vi "Configure Trigger (I2C - Address Or Data).vi"(0 "VISA resource name":refnum<visa-resource-name>, 1 "Trigger On (4:Address)":u16(ring)=4 items=["Address"=4, "Data"=5, "Address And Data"=6], 2 "Addressing Mode (0:7 Bit)":u16(ring) items=["7 Bit", "10 Bit"], 3 "Special Address (0:None)":u16(ring) items=["None", "Start", "General Call", "10 Bit"], 5 "Data Source":T2={"Data Source (0:Channel1)"=0, "Data Threshold (1.2V)"=1.2} {"Data Source (0:Channel1)" items=["Channel1", "Channel2", "Channel3", "Channel4"]}, 7 "Clock Source":T1={"Clock Source (1:Channel2) "=1, "Clock Threshold (1.2V)"=1.2} {"Clock Source (1:Channel2)" items=["Channel1", "Channel2", "Channel3", "Channel4"]}, 9 "Data Direction (0:Either)":u16(ring) items=["Either", "Read", "Write"], 11 "error in (no error)":errorcluster, 12 "Address Value":string, 13 "Data Start Position(0)":u16, 14 "Data Value":string) -> (4 "VISA resource name out":refnum<visa-resource-name>, 15 "error out":errorcluster)   [LabVIEW 2015, in "Tektronix 7000 Series.lvlib"]
doc: "Configures I2C trigger settings for an oscilloscope. A trigger occurs when an Inter-IC Control signal is found. This Vi is configure trigger on Address,Data, Address And Data\n\n<b>Note:</b>\nOnly DPO7000 series oscilloscopes Support this Trigger."
uses:
  <instrlib>/Tektronix 7000 Series/Tektronix 7000 Series.lvlib
panel:
  # "lsb"
  # "msb"
  # "msb"
  # "lsb"
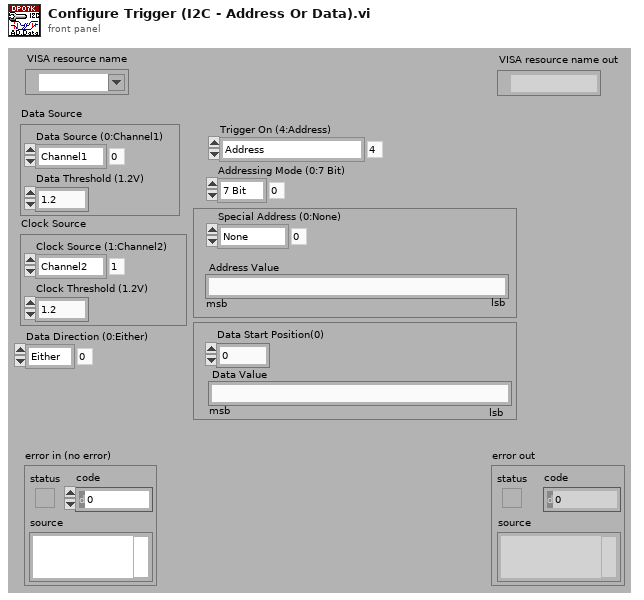
[diagram p1: front panel]
types:
  T1 = cluster{"Clock Source (1:Channel2) ":u16, "Clock Threshold (1.2V)":dbl}
  T2 = cluster{"Data Source (0:Channel1)":u16, "Data Threshold (1.2V)":dbl}
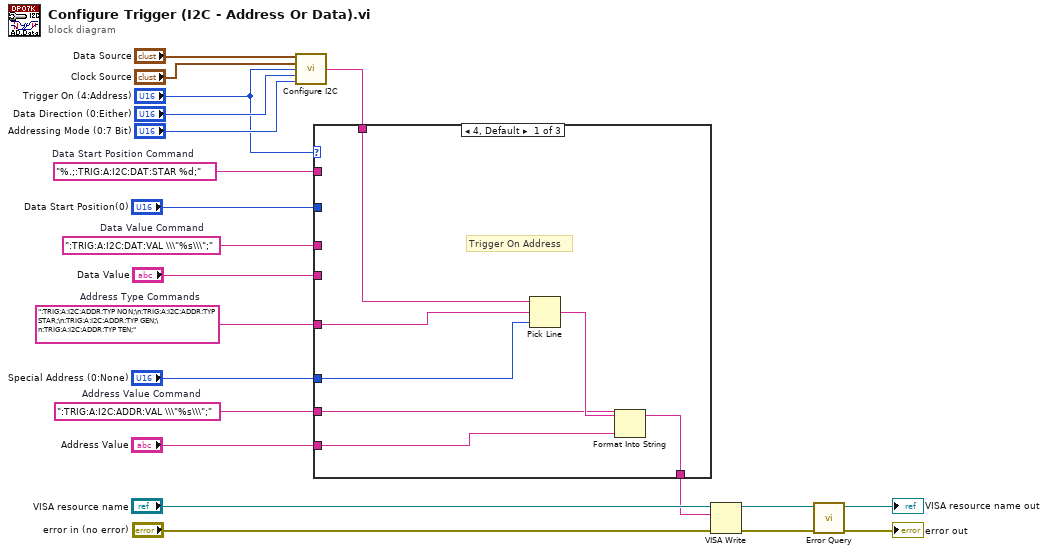
[diagram p0: block diagram]
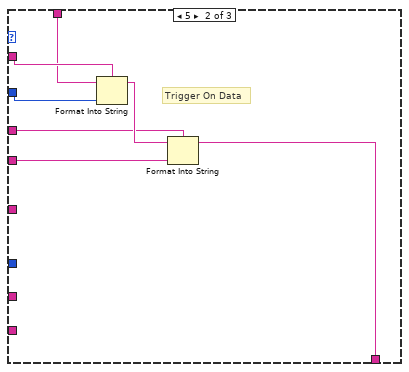
[diagram p2: hidden frame]
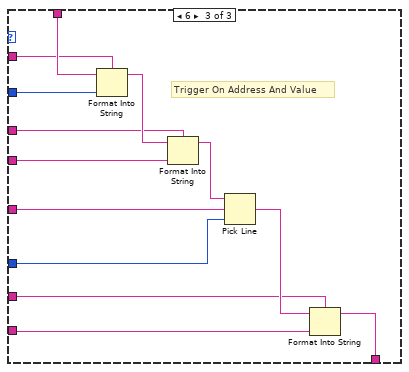
[diagram p3: hidden frame]
diagram:
  w8 = ":TRIG:A:I2C:ADDR:VAL \\\"%s\\\";"  # Address Value Command
  w11 = ":TRIG:A:I2C:ADDR:TYP NON;\n:TRIG:A:I2C:ADDR:TYP STAR;\n:TRIG:A:I2C:ADDR:TYP GEN;\n:TRIG:A:I2C:ADDR:TYP TEN;"  # Address Type Commands
  w15 = "%.;:TRIG:A:I2C:DAT:STAR %d;"  # Data Start Position Command
  w13 = ":TRIG:A:I2C:DAT:VAL \\\"%s\\\";"  # Data Value Command
  n1 = call <instrlib>:"Configure I2C.vi"("Data Source"="Data Source", "Clock Source"="Clock Source", "Trigger On (0:Start)"="Trigger On (4:Address)", "Data Direction (0:Either)"="Data Direction (0:Either)", "Addressing Mode (0:7 Bit)"="Addressing Mode (0:7 Bit)") -> ("Output String"=w16:string)  [unwired: 10 in]
  n2 = case shown="4, Default" "Trigger On (4:Address)" {
    tunnel: w16 -> [w27 w30 w48]
    tunnel: w15 -> [_ w32 w47]
    tunnel: "Data Start Position(0)" -> [_ w31 w46]
    tunnel: w13 -> [_ w33 w44]
    tunnel: "Data Value" -> [_ w34 w43]
    tunnel: w11 -> [w26 _ w42]
    tunnel: "Special Address (0:None)" -> [w25 _ w41]
    tunnel: "Address Value" -> [w23 _ w38]
    tunnel: w8 -> [w24 _ w37]
    tunnel: [w22 w29 w36] -> w4
    frame 4, Default {
      # "Trigger On Address"
      n3 = Pick Line(string ("")=w27, multi-line string=w26, line index=w25) -> (output string=w28:string)
      n4 = Format Into String(format string=w24, initial string=w28, w23) -> (resulting string=w22:string)  [unwired: 1 in, 1 out]
    }
    frame 5 {
      # "Trigger On Data"
      n5 = Format Into String(format string=w32, initial string=w30, w31) -> (resulting string=w35:string)  [unwired: 1 in, 1 out]
      n6 = Format Into String(format string=w33, initial string=w35, w34) -> (resulting string=w29:string)  [unwired: 1 in, 1 out]
    }
    frame 6 {
      # "Trigger On Address And Value"
      n7 = Format Into String(format string=w47, initial string=w48, w46) -> (resulting string=w45:string)  [unwired: 1 in, 1 out]
      n8 = Format Into String(format string=w44, initial string=w45, w43) -> (resulting string=w40:string)  [unwired: 1 in, 1 out]
      n9 = Pick Line(string ("")=w40, multi-line string=w42, line index=w41) -> (output string=w39:string)
      n10 = Format Into String(format string=w37, initial string=w39, w38) -> (resulting string=w36:string)  [unwired: 1 in, 1 out]
    }
  }
  n11 = VISA Write(VISA resource name="VISA resource name", write buffer=w4, error in (no error)="error in (no error)") -> (VISA resource name out=w6:refnum<visa-resource-name>, error out=w7:errorcluster)  [unwired: 1 out]
  n12 = call <instrlib>:"Error Query.vi"("error in (no error)"=w7, "VISA resource name"=w6) -> ("error out"=→"error out":errorcluster, "VISA resource name out"=→"VISA resource name out":refnum<visa-resource-name>)  [unwired: 6 in, 2 out]
